vi "Actor Core.vi"(8 "error in":errorcluster, 11 "Nested in":refnum<class "NXP.lvclass">) -> (0 "error out":errorcluster, 3 "Actor out":refnum<class "Actor.lvclass">)   [LabVIEW 2019, in "NXP.lvclass"]
doc: "(<B>Filename</B>: Actor Framework.lvlib:Actor.lvclass:Actor Core.vi)\n\nReceives messages to the actor, reacts to them, and initiates any error handling that may shut the actor down.\n\nDescendant classes may override this VI to append parallel tasks for the actor to complete while it handles messages. Overrides use the Call Parent Method node."
uses:
  NXP.lvclass
  C:/Program Files (x86)/National Instruments/LabVIEW 2019/vi.lib/ActorFramework/Actor/Actor.lvclass
  <vilib>/ActorFramework/Actor/Actor.lvclass
  <vilib>/ActorFramework/Actor/Actor.lvclass/Actor.ctl
  NXP.lvclass/NXP.ctl
  Serial Devices Messages/Get Data Msg/Get Data Msg.lvclass/Get Data Msg.ctl
  <vilib>/ActorFramework/Message Enqueuer/Message Enqueuer.lvclass/Message Enqueuer.ctl
  <vilib>/ActorFramework/Message Enqueuer/Enqueue.vi
  Serial Devices Messages/Get Data Msg/Get Data Msg.lvclass
  C:/Program Files (x86)/National Instruments/LabVIEW 2019/vi.lib/ActorFramework/Message/Message.lvclass
  <vilib>/ActorFramework/Message Priority Queue/Priority Enqueue.vi
  Serial Devices/Serial Devices.lvclass
  Serial Devices/Serial Devices.lvlib
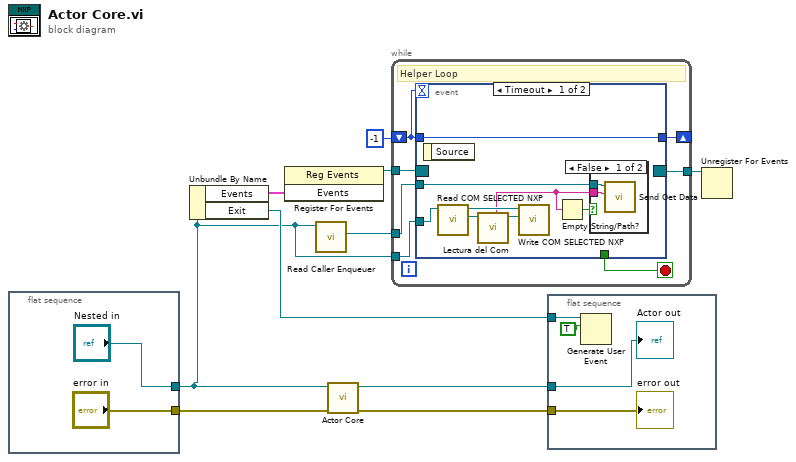
[diagram p0: block diagram]
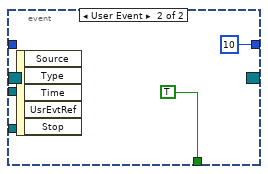
[diagram p3: hidden frame]
diagram:
  n1 = flat-sequence {
    tunnel: ["error in"] -> w7
    tunnel: ["Nested in"] -> w1
    frame #0 {
    }
  }
  n2 = Unbundle By Name(w1) -> ("Events"=w10:cluster{"Exit":refnum<user-event>}, "Exit"=w2:refnum<user-event>)
  n3 = register-events(w10) -> (reference out=w3:refnum<event-registration>)  [unwired: 2 in, 1 out]
  n4 = call <vilib>:"Read Caller Enqueuer.vi"("Actor"=w1) -> ("Caller Enqueuer"=w4:refnum<class "Message Enqueuer.lvclass">)  [unwired: 10 in]
  n5 = call-parent "Actor Core.vi"("error in"=w7, "Nested in"=w1) -> ("error out"=w8:errorcluster, "Actor out"=w9:refnum<class "Actor.lvclass">)  [unwired: 8 in]
  n6 = while {
    shift-right: [w19] -> _
    shift-left: -1 -> [w18]
    tunnel: w3 -> [w17]
    tunnel: [w16] -> w5
    tunnel: w4 -> [w14]
    tunnel: w1 -> [w13]
    stop <- w15 stop-if-true
    # "Helper Loop"
    n7 = event shown="[0] Timeout" {
      selector: w17 -> [_ _]
      dyn-events: [_ _] -> w16
      timeout: w18 -> [_ _]
      tunnel: w18 -> [w27 _]
      tunnel: [w27 10 ("f")] -> w19
      tunnel: [_ TRUE] -> w15
      tunnel: w14 -> [w26 _]
      tunnel: w13 -> [w22 _]
      event Timeout {
        n8 = event-data() -> ()  [unwired: 1 in, 1 out]
        n9 = call "Read COM SELECTED NXP.vi"("NXP in"=w22) -> ("COM SELECTED"=w25:refnum<visa-resource-name>, "NXP out"=w23:refnum<class "NXP.lvclass">)  [unwired: 8 in, 1 out]
        n10 = call "Lectura del Com.vi"("VISA Refnum in"=w25) -> ("Serial Response"=w21:string, "VISA resource name out"=w24:refnum<visa-resource-name>)  [unwired: 8 in, 1 out]
        n11 = call "Write COM SELECTED NXP.vi"("COM SELECTED"=w24, "NXP in"=w23) -> ()  [unwired: 8 in, 2 out]
        n12 = Empty String/Path?(string/path=w21) -> (empty?=w20:bool)
        n13 = case shown="False" w20 {
          tunnel: w26 -> [w29 _]
          tunnel: w21 -> [w28 _]
          frame False {
            n14 = call "Send Get Data.vi"("Data"=w28, "Message Enqueuer"=w29) -> ()  [unwired: 8 in, 2 out]
          }
          frame True {
          }
        }
      }
      event User Event {
        n15 = event-data() -> ()  [unwired: 1 in, 5 out]
      }
    }
  }
  n16 = flat-sequence {
    tunnel: w8 -> [w35]
    tunnel: w9 -> [w34]
    tunnel: w2 -> [w32]
    frame #0 {
      n17 = Generate User Event(user event=w32, event data cluster=TRUE ("event data")) -> ()  [unwired: 2 in, 2 out]
      "error out" <- w35
      "Actor out" <- w34
    }
  }
  n18 = Unregister For Events(event registration refnum=w5) -> ()  [unwired: 1 in, 1 out]
